vi "Tell Reply.vi"(4 "Priority":bool, 7 "Actor in":refnum<class "Actor.lvclass">, 10 "Msg":refnum<class "Msg.lvclass">) -> (0 "Error out":errorcluster)   [LabVIEW 2025, in "jettl.lvlib"]
uses:
  jettl.lvlib
  Msg/Msg.lvclass
  Actor/Actor.lvclass
  Teller/Teller.lvclass
  Msg Input/Msg Input.lvclass
  Attributes/Attributes.lvclass
  Error/Error.lvlib
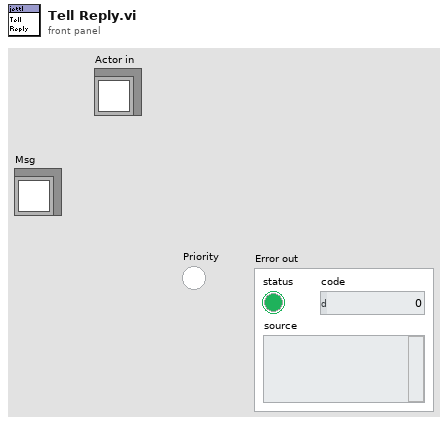
[diagram p1: front panel]
types:
  T1 = typedef "jettl.lvlib/Relation.ctl" = enum16{"Self", "Parent", "Child", "No Relation"}
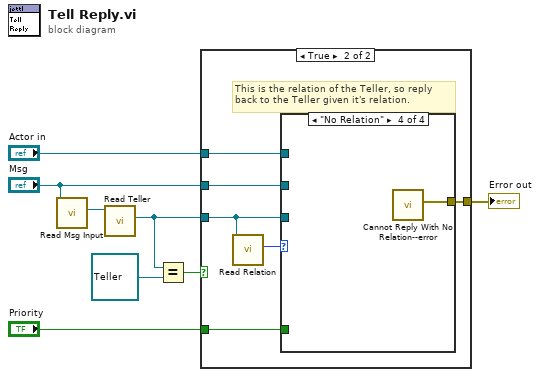
[diagram p0: block diagram]
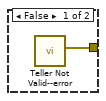
[diagram p2: hidden frame]
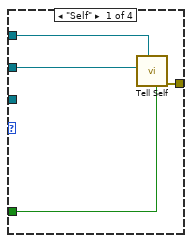
[diagram p3: hidden frame]
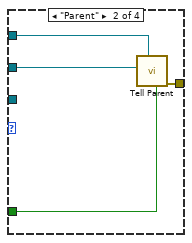
[diagram p4: hidden frame]
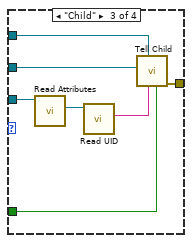
[diagram p5: hidden frame]
diagram:
  n1 = call-dynamic "Read Msg Input.vi"("Msg in"="Msg") -> ("Msg Input"=w3:refnum<class "Msg Input.lvclass">)  [unwired: 10 in]
  n2 = call-dynamic "Read Teller.vi"("Msg Input in"=w3) -> ("Teller"=w1:refnum<class "Teller.lvclass">)  [unwired: 10 in]
  n3 = Equal?(x=w1, y=refnum<class "Teller.lvclass"> refnum ("Sender")) -> (x = y?=w6:bool)
  n4 = case shown="True" w6 {
    tunnel: "Actor in" -> [_ w15]
    tunnel: "Msg" -> [_ w14]
    tunnel: "Priority" -> [_ w13]
    tunnel: w1 -> [_ w12]
    tunnel: [w9 w10] -> w7
    frame False {
      n5 = call "Teller Not Valid--error.vi"() -> ("Error"=w9:errorcluster)  [unwired: 11 in]
    }
    frame True {
      # "This is the relation of the Teller, so reply back to the Teller given it's relation."
      n6 = call-dynamic "Read Relation.vi"("Teller in"=w12) -> ("Relation"=w11:T1)  [unwired: 10 in]
      n7 = case shown="\"No Relation\"" w11 {
        tunnel: w15 -> [w19 w23 w28 _]
        tunnel: w14 -> [w18 w22 w27 _]
        tunnel: w13 -> [w17 w21 w25 _]
        tunnel: w12 -> [_ _ w30 _]
        tunnel: [w16 w20 w24 w31] -> w10
        frame "Self" {
          n8 = call "Tell Self.vi"("Priority"=w17, "Actor in"=w19, "Msg"=w18) -> ("Error out"=w16:errorcluster)  [unwired: 8 in]
        }
        frame "Parent" {
          n9 = call "Tell Parent.vi"("Priority"=w21, "Actor in"=w23, "Msg"=w22) -> ("Error out"=w20:errorcluster)  [unwired: 8 in]
        }
        frame "Child" {
          n10 = call-dynamic "Read Attributes.vi"("Teller in"=w30) -> ("Attributes"=w29:refnum<class "Attributes.lvclass">)  [unwired: 10 in]
          n11 = call-dynamic "Read UID.vi"("Attributes in"=w29) -> ("UID"=w26:string)  [unwired: 10 in]
          n12 = call "Tell Child.vi"("Priority"=w25, "UID"=w26, "Actor in"=w28, "Msg"=w27) -> ("Error out"=w24:errorcluster)  [unwired: 7 in]
        }
        frame "No Relation" {
          n13 = call "Cannot Reply With No Relation--error.vi"() -> ("Error"=w31:errorcluster)  [unwired: 11 in]
        }
      }
    }
  }
  "Error out" <- w7
